vi "getTopEnumNameAndLiteral.vi"(8 "error in (no error)":errorcluster, 10 "IDLConstants":string, 11 "Enumeration in":refnum<class "Enumeration.lvclass">) -> (0 "error out":errorcluster, 1 "enumerationLiteral":string, 2 "enumName":string, 3 "Enumeration out":refnum<class "Enumeration.lvclass">, 4 "endOfString":bool, 5 "restOfString":string, 6 "noMatch":bool)   [LabVIEW 2016, in "Enumeration.lvclass"]
uses:
  Enumeration.lvclass
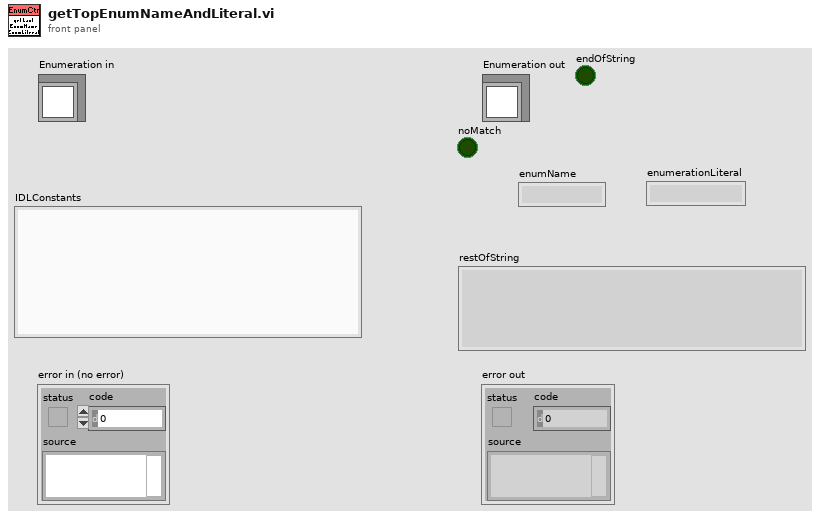
[diagram p1: front panel]
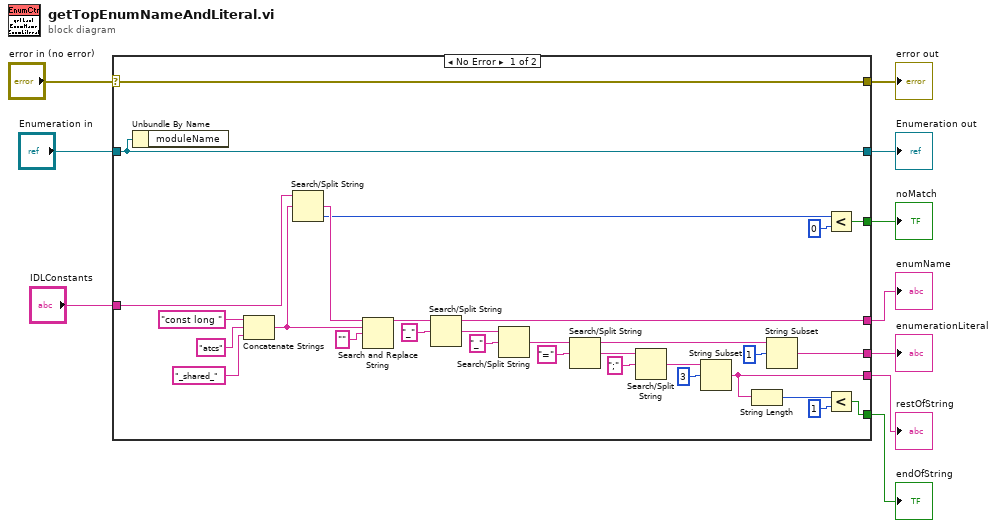
[diagram p0: block diagram]
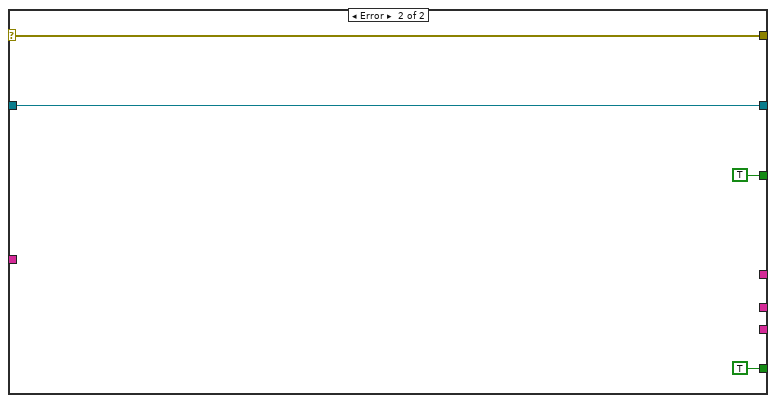
[diagram p2: hidden frame]
diagram:
  n1 = case shown="No Error" "error in (no error)" {
    selector: "error in (no error)" -> [w40 w44]
    tunnel: [w40 w44] -> w9
    tunnel: [w30 w43] -> w8
    tunnel: "Enumeration in" -> [w30 w43]
    tunnel: [w36 _] -> w7
    tunnel: "IDLConstants" -> [w31 _]
    tunnel: [w17 _] -> w4
    tunnel: [w23 _] -> w3
    tunnel: [w14 TRUE] -> w2
    tunnel: [w11 TRUE] -> w1
    frame No Error {
      n2 = Unbundle By Name(w30) -> ()  [unwired: 1 out]
      n3 = Concatenate Strings("const long ", "atcs" ("string"), "_shared_" ("string")) -> (w34:string)
      n4 = Search/Split String(string=w31, search string/char (-)=w34) -> (match + rest of string=w35:string, offset of match=w13:i32)  [unwired: 1 in, 1 out]
      n5 = Search and Replace String(input string=w35, search string=w34, replace string="" ("replace string (\"\")")) -> (result string=w32:string)  [unwired: 5 in, 3 out]
      n6 = Search/Split String(string=w32, search string/char (-)="_") -> (substring before match=w36:string, match + rest of string=w29:string)  [unwired: 1 in, 1 out]
      n7 = Search/Split String(string=w29, search string/char (-)="_") -> (match + rest of string=w26:string)  [unwired: 1 in, 2 out]
      n8 = Search/Split String(string=w26, search string/char (-)="=") -> (substring before match=w25:string, match + rest of string=w22:string)  [unwired: 1 in, 1 out]
      n9 = Search/Split String(string=w22, search string/char (-)=";") -> (match + rest of string=w19:string)  [unwired: 1 in, 2 out]
      n10 = String Subset(string=w19, offset (0)=3) -> (substring=w17:string)  [unwired: 1 in]
      n11 = String Length(string=w17) -> (length=w16:i32)
      n12 = String Subset(string=w25, offset (0)=1) -> (substring=w23:string)  [unwired: 1 in]
      n13 = Less?(x=w13, y=0) -> (x < y?=w11:bool)
      n14 = Less?(x=w16, y=1) -> (x < y?=w14:bool)
    }
    frame Error {
    }
  }
  "error out" <- w9
  "Enumeration out" <- w8
  "enumName" <- w7
  "enumerationLiteral" <- w3
  "restOfString" <- w4
  "endOfString" <- w2
  "noMatch" <- w1
